vi "initialize.vi"(8 "error in (no error)":errorcluster, 9 "Optometer cfg file":path=path "C:/Gigahertz-Optik/config/TR9600MPEconfig.gdf", 10 "deviceName":string="TR9600_57976", 11 "password":string="ds,94ms2") -> (0 "error out":errorcluster, 2 "function return":i32, 3 "handle":i32)   [LabVIEW 2018]
uses:
  <userlib>/Gigahertz-Optik/GOMDTR9600/GOMDTR9600.lvlib
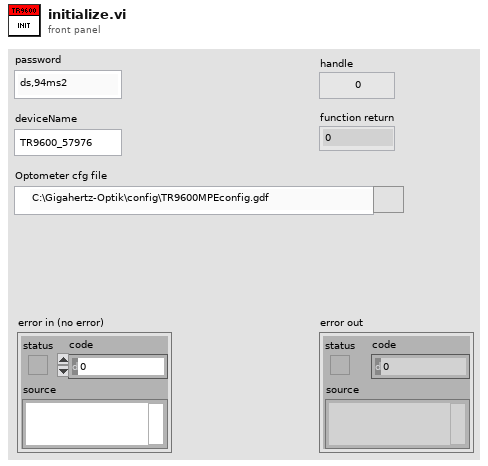
[diagram p1: front panel]
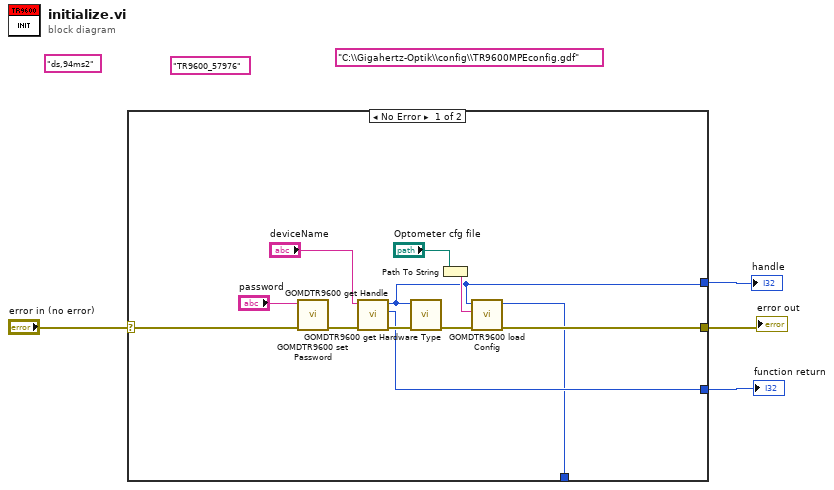
[diagram p0: block diagram]
diagram:
  (unwired) "C:\\Gigahertz-Optik\\config\\TR9600MPEconfig.gdf" ("value")
  (unwired) "TR9600_57976" ("deviceName")
  (unwired) "ds,94ms2" ("value")
  n1 = case shown="No Error" "error in (no error)" {
    selector: "error in (no error)" -> [w9 w17]
    tunnel: [w10 w17] -> w4
    tunnel: [w7 _] -> w2
    tunnel: [w6 _] -> w1
    tunnel: [w5 _] -> _
    frame No Error {
      n2 = call <userlib>:"GOMDTR9600 set Password.vi"("error in (no error)"=w9, "value"="password") -> ("error out"=w16:errorcluster)  [unwired: 8 in, 1 out]
      n3 = call <userlib>:"GOMDTR9600 get Handle.vi"("error in (no error)"=w16, "deviceName"="deviceName") -> ("error out"=w15:errorcluster, "function return"=w6:i32, "handle"=w7:i32)  [unwired: 7 in]
      n4 = call <userlib>:"GOMDTR9600 get Hardware Type.vi"("error in (no error)"=w15, "handle"=w7) -> ("error out"=w14:errorcluster)  [unwired: 7 in, 2 out]
      n5 = Path To String(path="Optometer cfg file") -> (string=w8:string)
      n6 = call <userlib>:"GOMDTR9600 load Config.vi"("error in (no error)"=w14, "filename"=w8, "handle"=w7) -> ("error out"=w10:errorcluster, "function return"=w5:i32)  [unwired: 7 in]
    }
    frame Error {
    }
  }
  "error out" <- w4
  "handle" <- w2
  "function return" <- w1
